vi "xml-rpc example.vi"() -> ()   [LabVIEW 2010]
uses:
  <vilib>/httpClient/POSTBuffer.vi
  <vilib>/httpClient/LabVIEWHTTPClient.lvlib
panel:
  in  "Parameters":i32[](array[numeric])=[44]
  in  "method name":string="examples.getStateName"
  out "XML-RPC String":string
  in  "URL":string="phpxmlrpc.sourceforge.net/server.php"
  out "response body":string
  out "response header":string
  # "Goto http://phpxmlrpc.sourceforge.net/server.php in your webbrowser for doucmentation of the server"
  # "This example only supports \nnumeric parameters for now"
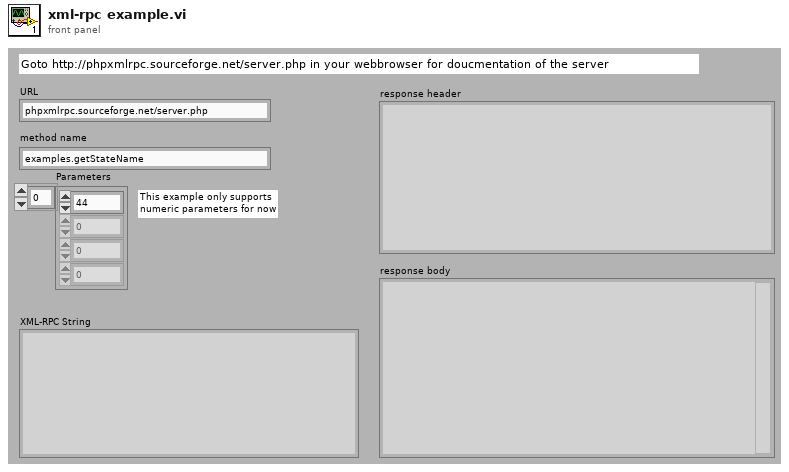
[diagram p1: front panel]
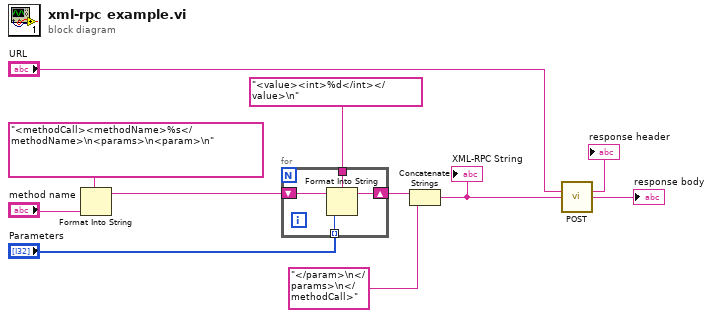
[diagram p0: block diagram]
diagram:
  n1 = Format Into String(format string="<methodCall><methodName>%s</methodName>\n<params>\n<param>\n" ("XML-RPS String"), "method name") -> (resulting string=w6:string)  [unwired: 2 in, 1 out]
  n2 = for {
    shift-right: [w14] -> w2
    shift-left: w6 -> [w15]
    tunnel: "Parameters" -> [w13] mode=indexing
    tunnel: "<value><int>%d</int></value>\n" ("XML-RPS String") -> [w12]
    n3 = Format Into String(format string=w12, initial string=w15, w13) -> (resulting string=w14:string)  [unwired: 1 in, 1 out]
  }
  n4 = Concatenate Strings(w2, "</param>\n</params>\n</methodCall>" ("XML-RPS String")) -> (w1:string)
  "XML-RPC String" <- w1
  n5 = call-poly <vilib>:"POST.vi"("URL"="URL", "data"=w1) -> ("headers"=→"response header":string, "body"=→"response body":string)  [unwired: 10 in, 2 out]
